vi "Single Register.vi"() -> ()   [LabVIEW 2018]
uses:
  api/Failure Information.ctl
  api/Log Record.ctl
  api/logger_class/Internal Log Levels.ctl
  api/GLog.lvlib
panel:
  out "error out":errorcluster
  out "failures info":T1[](array[typedef]) {"Log Record"."timestamp" format="%<%x %.3X>T"}
  out "register test":bool
  # "Locals"
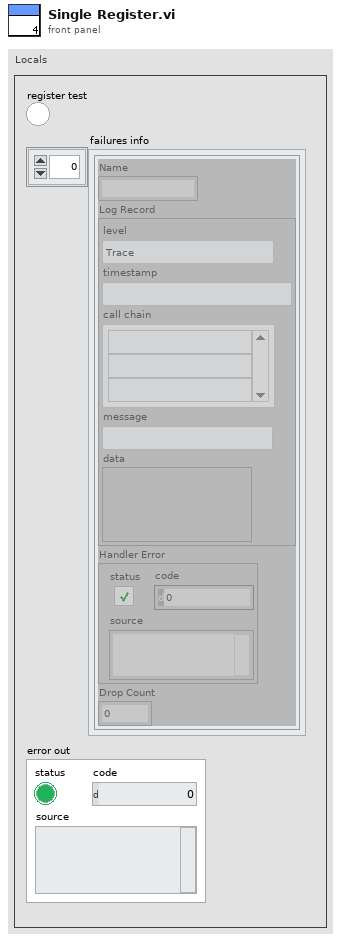
[diagram p1: front panel]
types:
  T1 = typedef "GLog.lvlib/Failure Information.ctl" = cluster{"Name":string, "Log Record":T2, "Handler Error":errorcluster, "Drop Count":u32}
  T2 = typedef "GLog.lvlib/Log Record.ctl" = cluster{"level":T3, "timestamp":timestamp, "call chain":string[], "message":string, "data":variant}
  T3 = typedef "GLog.lvlib/Internal Log Levels.ctl" = enum16{"Trace", "Debug", "Info", "Warning", "Error", "Critical", "Internal"}
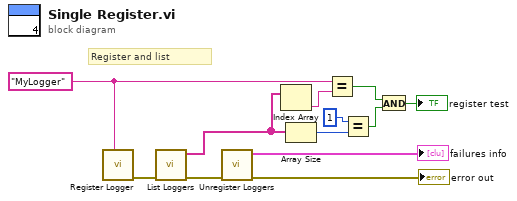
[diagram p0: block diagram]
diagram:
  w6 = "MyLogger" ("name")
  # "Register and list"
  n1 = call "Register Logger.vi"("name (\"Default\")"=w6) -> ("error out"=w5:errorcluster)  [unwired: 10 in]
  n2 = call "List Loggers.vi"("error in (no error)"=w5) -> ("error out"=w3:errorcluster, "registered loggers"=w4:string[])  [unwired: 9 in]
  n3 = call "Unregister Loggers.vi"("error in (no error)"=w3) -> ("error out"=→"error out":errorcluster, "failures info"=→"failures info":T1[])  [unwired: 9 in]
  n4 = Index Array(array=w4) -> (element=w10:string)  [unwired: 1 in]
  n5 = Array Size(array=w4) -> (size(s)=w12:i32)
  n6 = Equal?(x=w6, y=w10) -> (x = y?=w9:bool)
  n7 = Equal?(x=1, y=w12) -> (x = y?=w8:bool)
  n8 = And(x=w9, y=w8) -> (x .and. y?=→"register test":bool)
